vi "Set Color Transparent.vi"(0 "Controls[]":refnum<vi>[](array[refnum])) -> ()   [LabVIEW 2017, in "GUI.lvlib"]
uses:
  GUI.lvlib
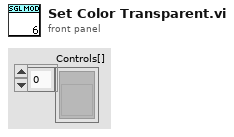
[diagram p1: front panel]
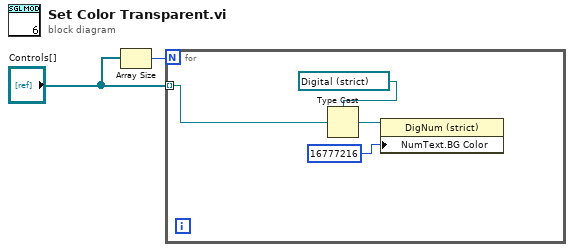
[diagram p0: block diagram]
diagram:
  n1 = Array Size(array="Controls[]") -> (size(s)=w2:i32)
  n2 = for {
    N: w2 -> [_]
    tunnel: "Controls[]" -> [w4] mode=indexing
    n3 = Type Cast(type=refnum<vi> refnum ("reference"), x=w4) -> (*(type *) &x=w6:refnum<vi>)
    n4 = property on="Property Node" class="DigNum (strict)"(reference=w6, "NumText.BG Color"=u32 16777216) -> ()  [unwired: 1 in, 2 out]
  }
